vi "HMI Respirador - copia.vi"() -> ()   [LabVIEW 2019]
uses:
  <vilib>/Instr/_visa.llb/VISA Configure Serial Port (Instr).vi
panel:
  out "Pulmones":dbl(ring)
  out "Waveform Chart":dynamicdata(graph)
  out "V. Espir.":bool
  out "V.Aspir":bool
  out "Trama de Datos":string
  out "Meter":i32(knob) scale=0.0..300.0
  out "Ventilador":bool
  out "TUBERIA EXHALACION":i32(slide)
  out "TUBERIA INHALACION":i32(slide) scale=0.0..115.0
  in  "stop":bool
  out "Velocidad Motor  R.P.M":i32
  out "Presion Entregada":i32
  in  "Tiempo PEEP":u16
  out "read buffer":string
  out "Boolean":bool
  in  "Guardar Config":bool
  in  "Iniciar":bool
  in  "Puerto Comunicación":refnum<visa-resource-name>
  in  "Presión Maxima":u8
  in  "PEEP (pres. esp.)":u8
  in  "Tiempo Anspiracion":u16
  in  "Turbina %":u8
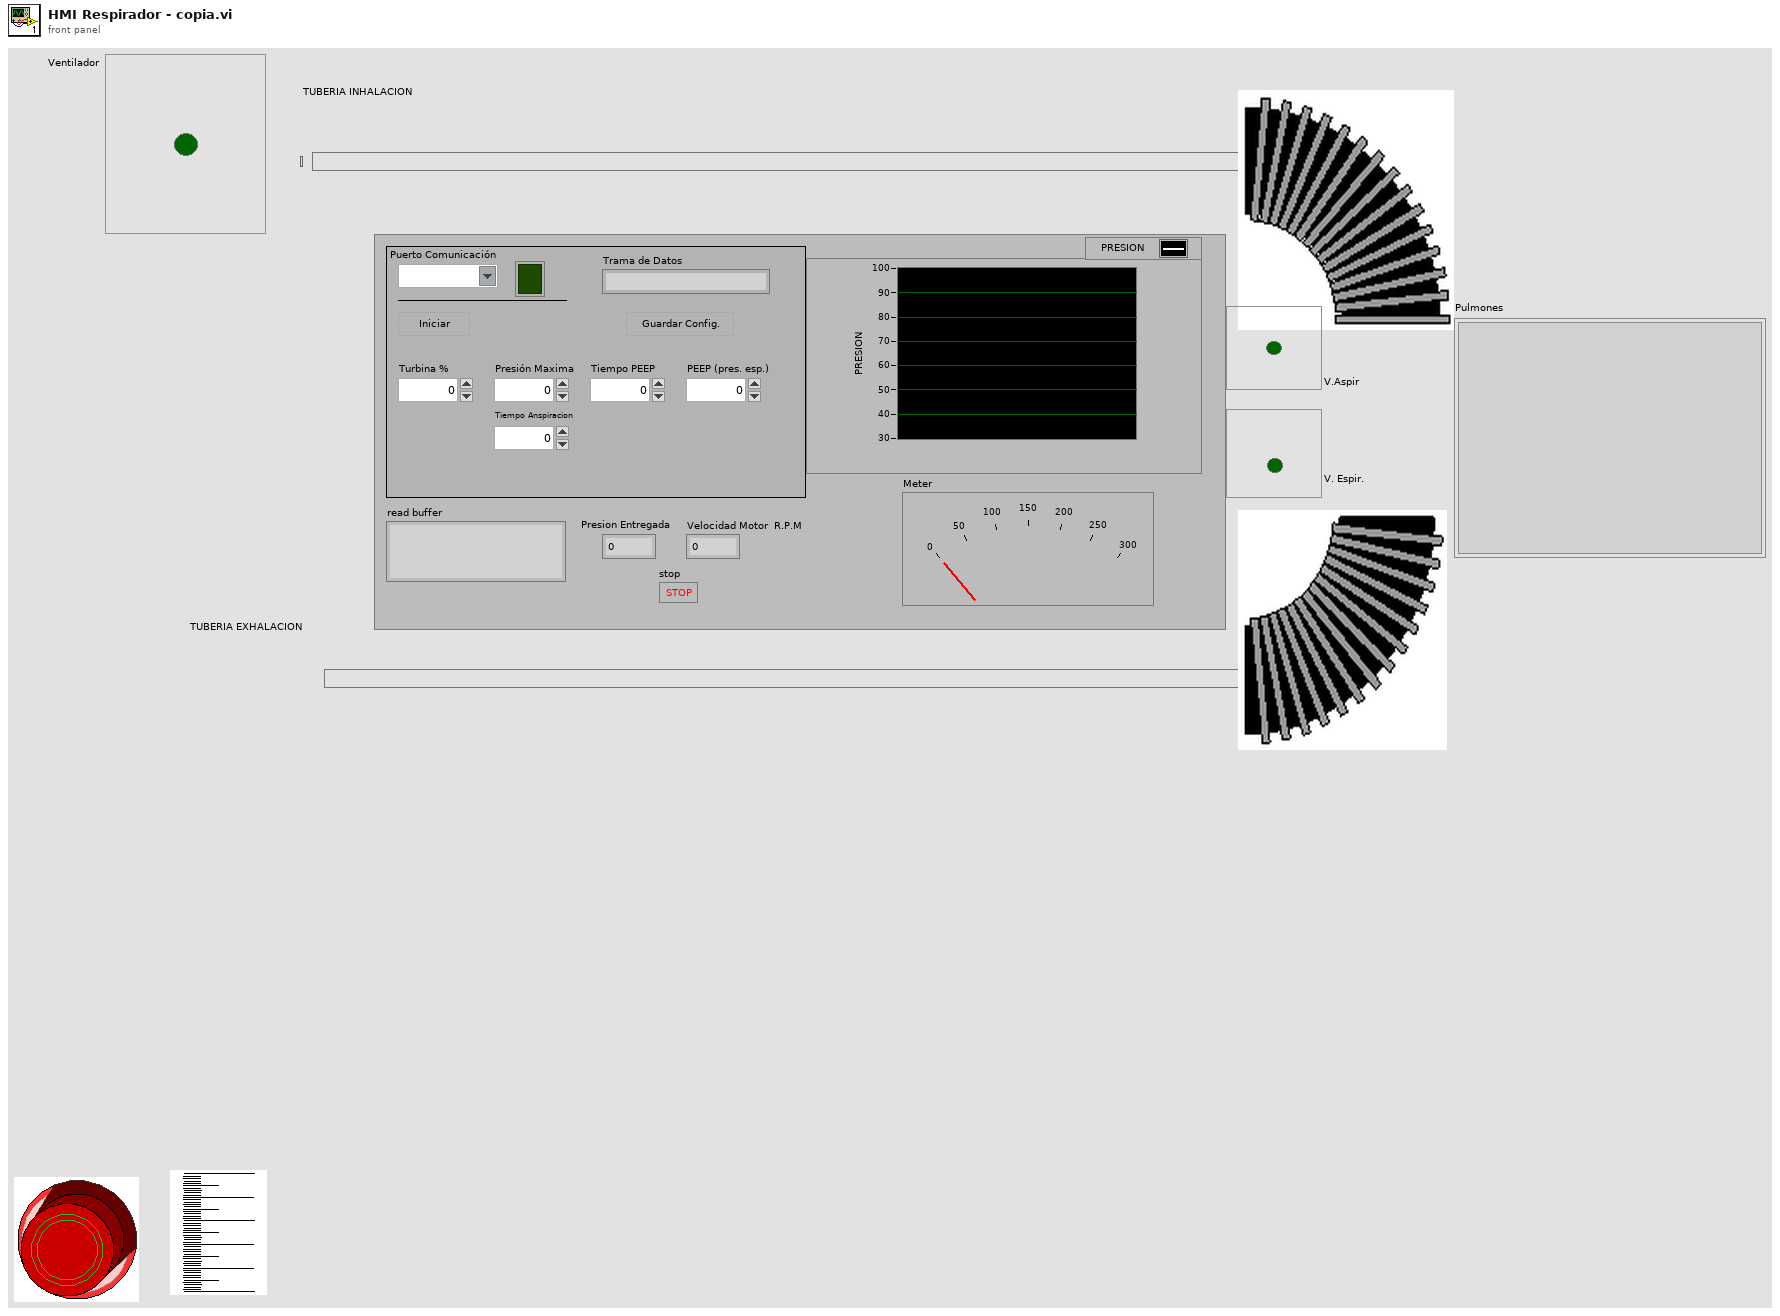
[diagram p1: front panel]
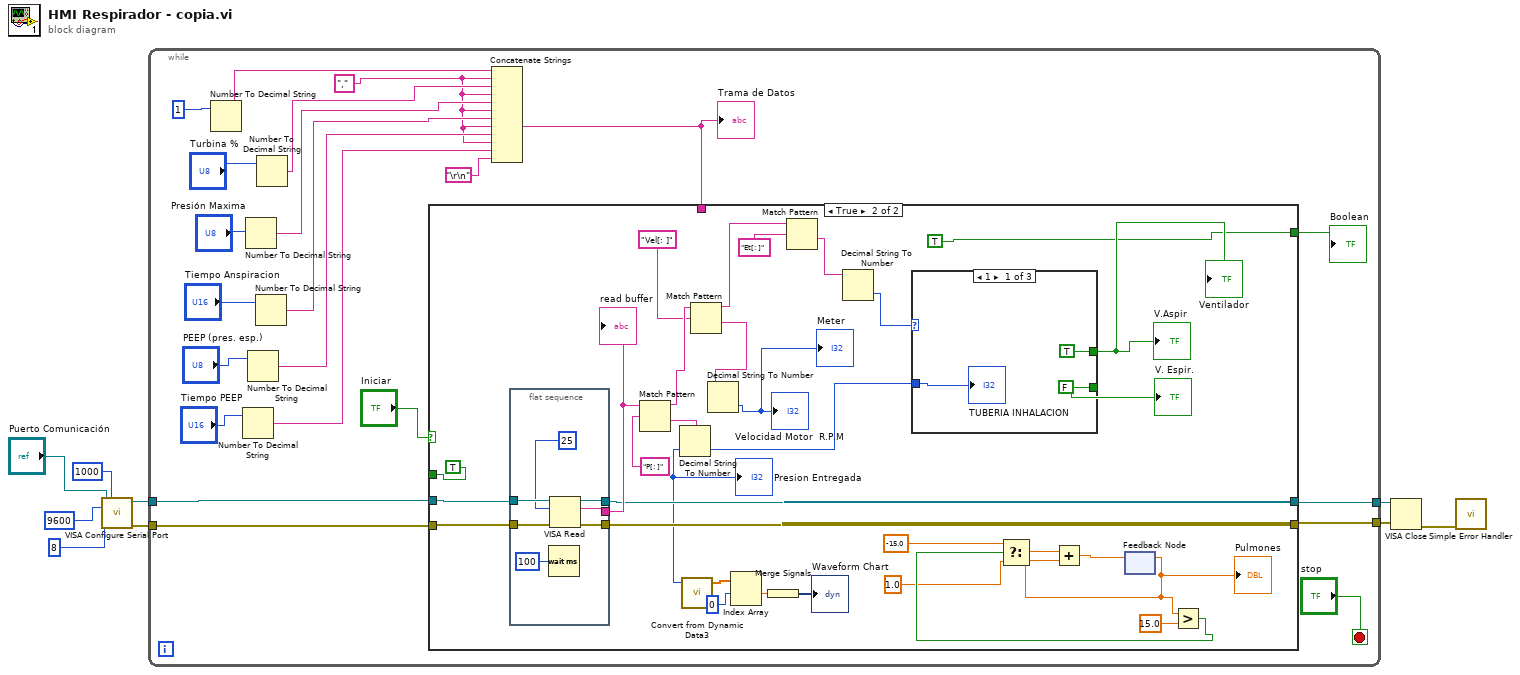
[diagram p0: block diagram]
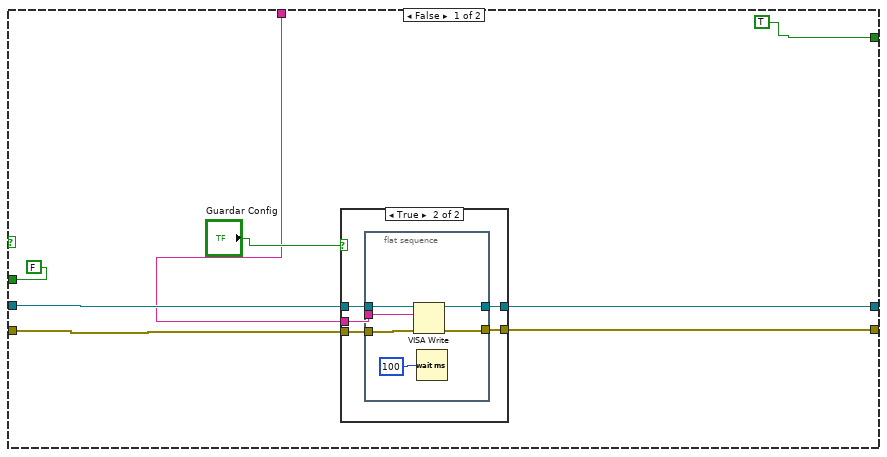
[diagram p2: hidden frame]
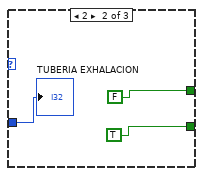
[diagram p4: hidden frame]
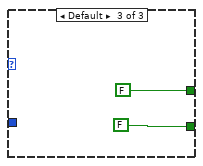
[diagram p5: hidden frame]
diagram:
  n1 = call-poly "VISA Configure Serial Port"("VISA resource name"="Puerto Comunicación", "timeout (10sec)"=u32 1000, "baud rate (9600)"=u32 9600, "data bits (8)"=u16 8) -> ("VISA resource name out"=w8:refnum<visa-resource-name>, "error out"=w7:errorcluster)  [unwired: 5 in, 5 out]
  n2 = while {
    tunnel: w8 -> [w30]
    tunnel: w7 -> [w31]
    tunnel: [w29] -> w4
    tunnel: [w28] -> w3
    stop <- "stop" stop-if-true
    w19 = ","
    n3 = Number To Decimal String(number=1) -> (decimal integer string=w24:string)  [unwired: 1 in]
    n4 = Number To Decimal String(number="Tiempo PEEP") -> (decimal integer string=w18:string)  [unwired: 1 in]
    n5 = Number To Decimal String(number="Presión Maxima") -> (decimal integer string=w22:string)  [unwired: 1 in]
    n6 = Number To Decimal String(number="PEEP (pres. esp.)") -> (decimal integer string=w20:string)  [unwired: 1 in]
    n7 = Number To Decimal String(number="Tiempo Anspiracion") -> (decimal integer string=w21:string)  [unwired: 1 in]
    n8 = Number To Decimal String(number="Turbina %") -> (decimal integer string=w23:string)  [unwired: 1 in]
    n9 = Concatenate Strings(w24, w19, w23, w19, w22, w19, w21, w19, w20, w19, w18, "\r\n") -> (w11:string)
    "Trama de Datos" <- w11
    n10 = case shown="True" "Iniciar" {
      tunnel: w30 -> [w37 w66]
      tunnel: w31 -> [w36 w67]
      tunnel: [w39 w69] -> w29
      tunnel: [w38 w68] -> w28
      tunnel: [TRUE TRUE] -> w17
      tunnel: w11 -> [w34 _]
      tunnel: [FALSE TRUE] -> _
      frame False {
        n11 = case shown="True" "Guardar Config" {
          tunnel: w34 -> [_ w46]
          tunnel: [w40 w45] -> w39
          tunnel: [w41 w44] -> w38
          tunnel: w37 -> [w40 w43]
          tunnel: w36 -> [w41 w42]
          frame False {
          }
          frame True {
            n12 = flat-sequence {
              tunnel: w43 -> [w52]
              tunnel: w42 -> [w51]
              tunnel: w46 -> [w50]
              tunnel: [w49] -> w45
              tunnel: [w48] -> w44
              frame #0 {
                n13 = VISA Write(VISA resource name=w52, write buffer=w50, error in (no error)=w51) -> (VISA resource name out=w49:refnum<visa-resource-name>, error out=w48:errorcluster)  [unwired: 1 out]
                n14 = Wait (ms)(milliseconds to wait=u32 100) -> ()  [unwired: 1 out]
              }
            }
          }
        }
      }
      frame True {
        n15 = flat-sequence {
          tunnel: w66 -> [w98]
          tunnel: w67 -> [w97]
          tunnel: [w96] -> w69
          tunnel: [w95] -> w68
          tunnel: [w94] -> w73
          frame #0 {
            n16 = Wait (ms)(milliseconds to wait=u32 100) -> ()  [unwired: 1 out]
            n17 = VISA Read(VISA resource name=w98, byte count=u32 25, error in (no error)=w97) -> (VISA resource name out=w96:refnum<visa-resource-name>, read buffer=w94:string, error out=w95:errorcluster)  [unwired: 1 out]
          }
        }
        n18 = Match Pattern(string=w73, regular expression="P[: ]") -> (before substring=w74:string, after substring=w71:string)  [unwired: 1 in, 2 out]
        n19 = Decimal String To Number(string=w71) -> (number=w62:i32)  [unwired: 2 in, 1 out]
        "Presion Entregada" <- w62
        n20 = call "Convert from Dynamic Data3"("Dynamic Data Type"=w62) -> ("Array"=w77:dbl[])  [unwired: 3 in]
        n21 = Match Pattern(string=w74, regular expression="Vel[: ]") -> (before substring=w75:string, after substring=w80:string)  [unwired: 1 in, 2 out]
        n22 = Decimal String To Number(string=w80) -> (number=→"Velocidad Motor  R.P.M" →"Meter":i32)  [unwired: 2 in, 1 out]
        n23 = Index Array(array=w77, index #1=0 ("index")) -> (element #1=w78:dbl)  [unwired: 1 in, 1 out]
        n24 = Merge Signals(w78) -> (→"Waveform Chart":dynamicdata)
        n25 = Match Pattern(string=w75, regular expression="Et[: ]") -> (after substring=w64:string)  [unwired: 1 in, 3 out]
        n26 = Decimal String To Number(string=w64) -> (number=w63:i32)  [unwired: 2 in, 1 out]
        n27 = case shown="1" w63 {
          tunnel: [TRUE FALSE FALSE] -> w82
          tunnel: [FALSE TRUE FALSE] -> w81
          tunnel: w62 -> [w85 w87 _]
          frame 1 {
            "TUBERIA INHALACION" <- w85
          }
          frame 2 {
            "TUBERIA EXHALACION" <- w87
          }
          frame Default {
          }
        }
        "Ventilador" <- w82
        "V.Aspir" <- w82
        "V. Espir." <- w81
        n28 = feedback #1() -> (w60:dbl)  [unwired: 1 in]
        "Pulmones" <- w60
        n29 = Greater?(x=w60, y=15.0) -> (0:w59:bool)
        n30 = Select(t=-15.0 ("y"), s=w59, f=1.0) -> (s? t:f=w58:dbl)
        n31 = Add(x=w58, y=w60) -> (x+y=w54:dbl)
        n32 = feedback-in #1(w54) -> ()
        "read buffer" <- w73
      }
    }
    "Boolean" <- w17
  }
  n33 = VISA Close(VISA resource name=w4, error in (no error)=w3) -> (error out=w9:errorcluster)
  n34 = call <vilib>:"Simple Error Handler.vi"("error in (no error)"=w9) -> ()  [unwired: 1 in, 8 out]
